vi "ttm_variableSaver_poller.vi"   [LabVIEW 2010]
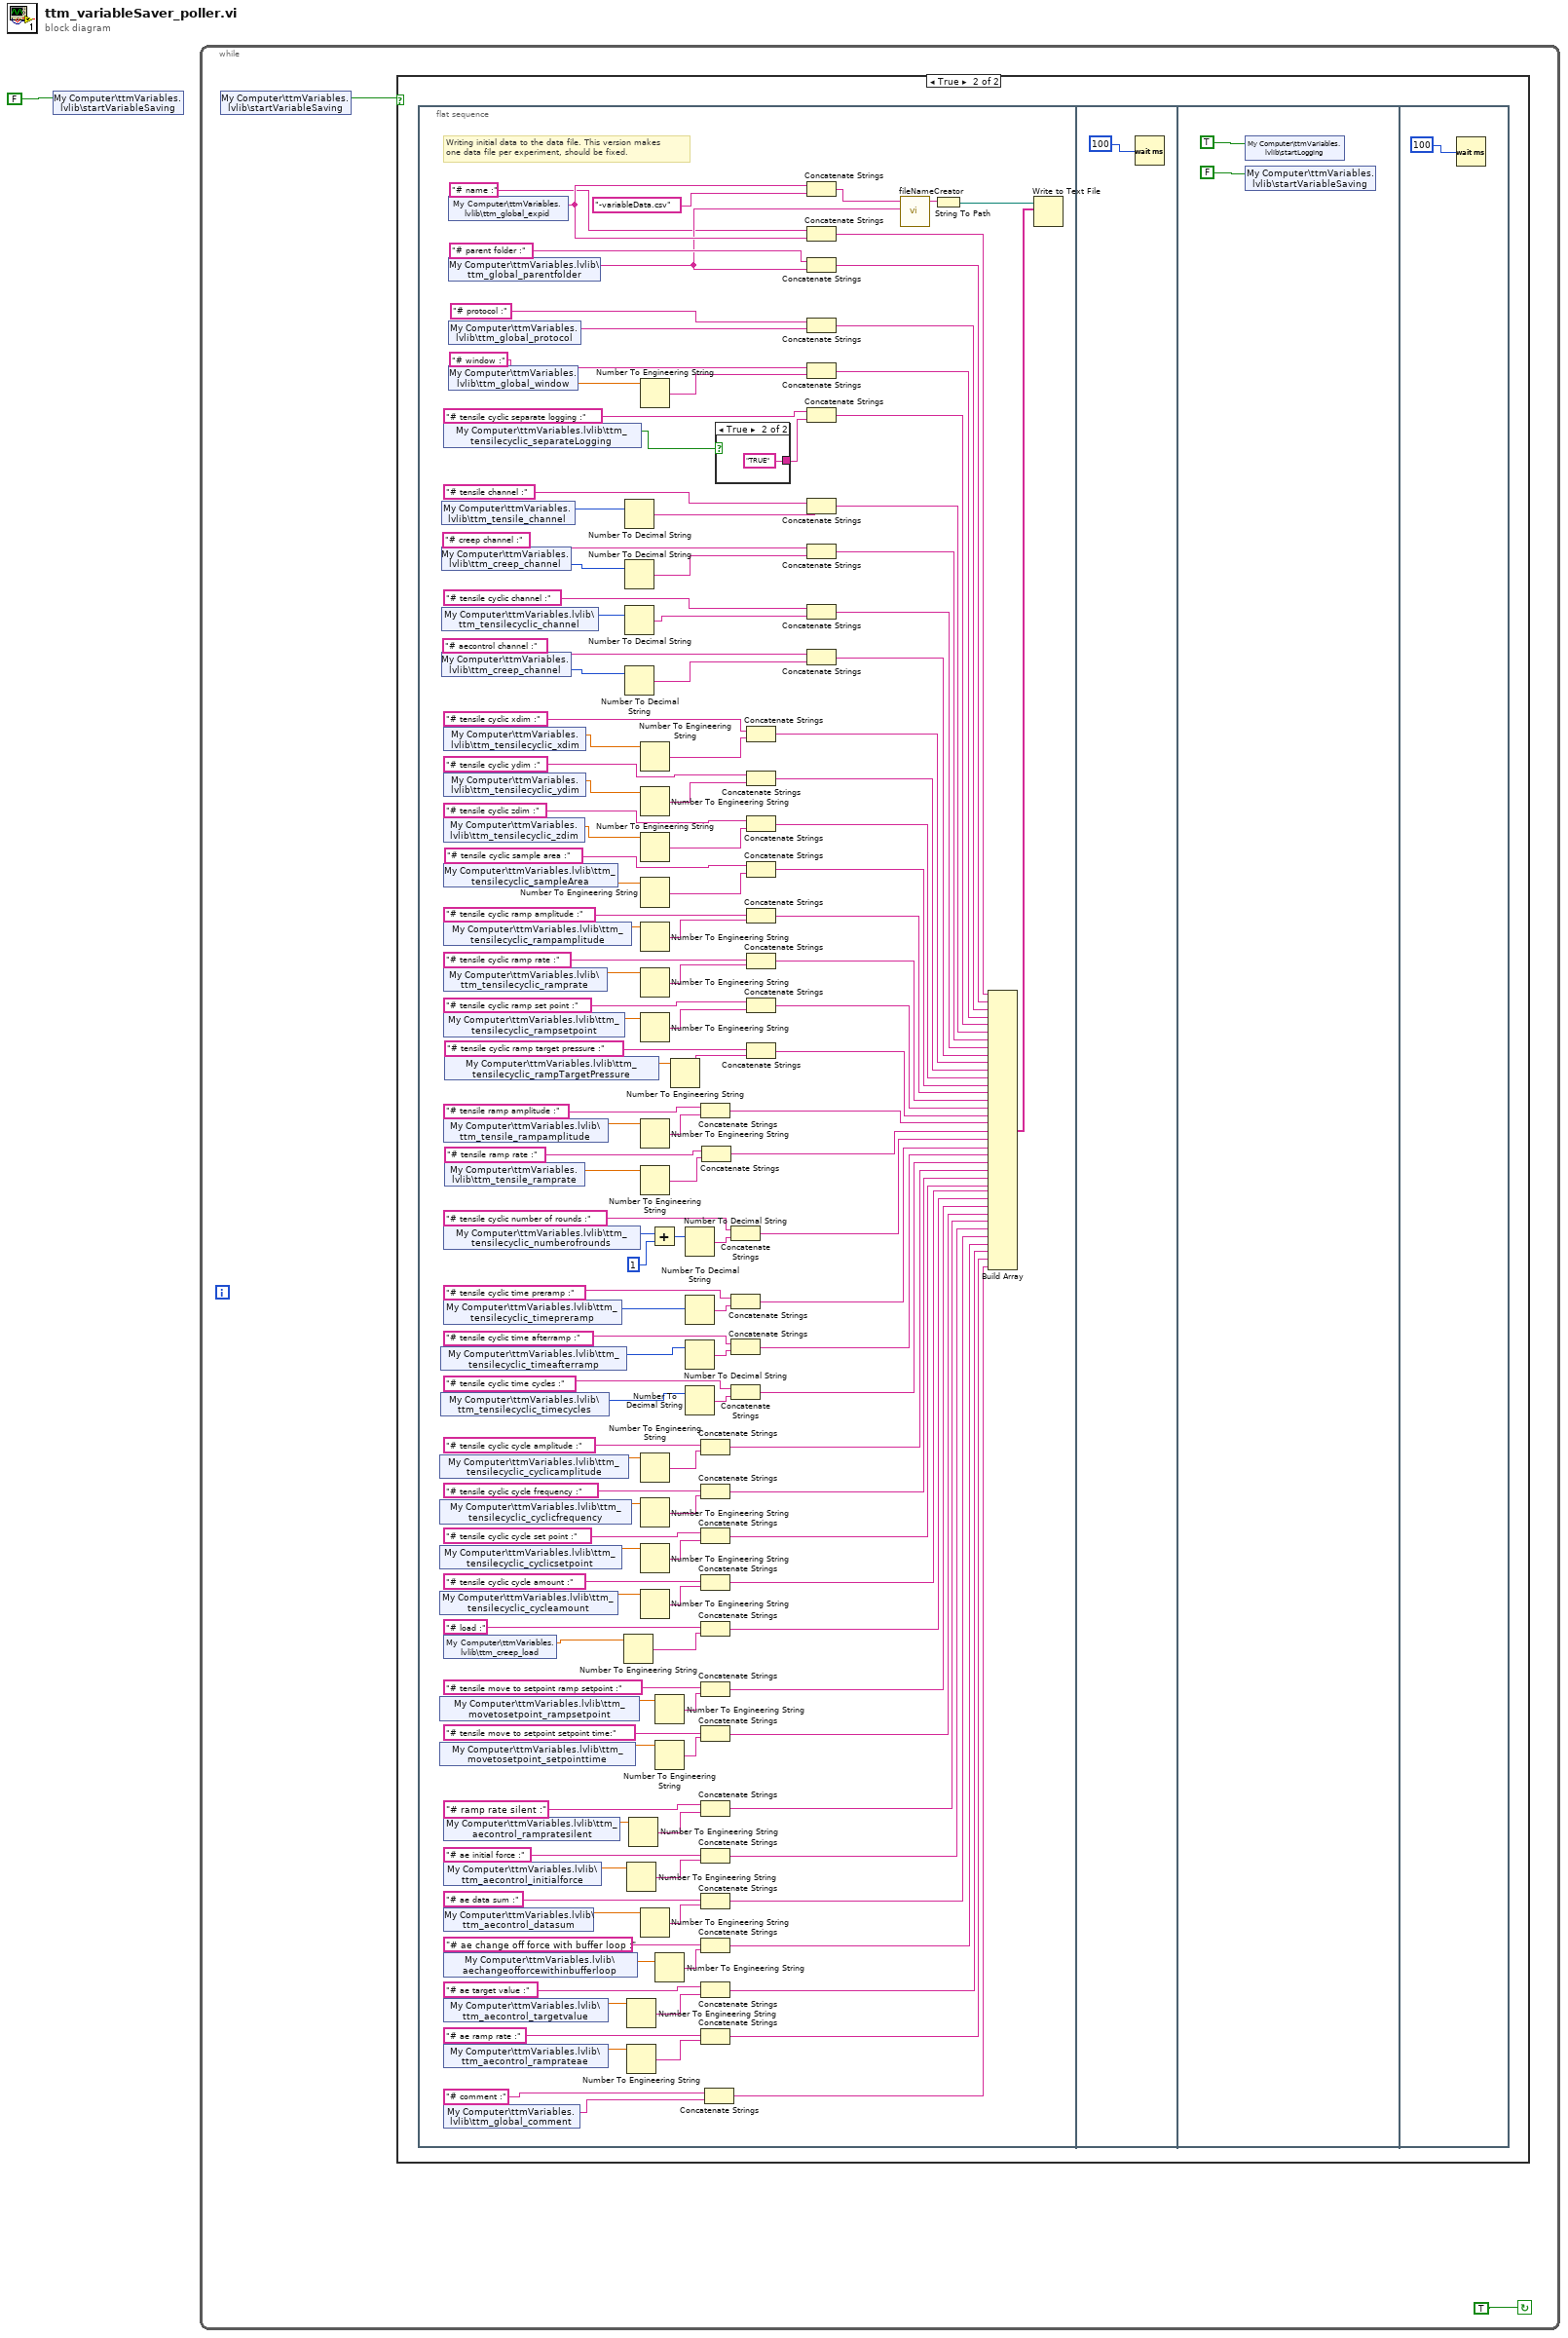
[diagram p0: block diagram]
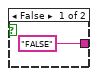
[diagram p3: hidden frame]
diagram:
  n1 = shared-variable "My Computer\\ttmVariables.lvlib\\startVariableSaving"(FALSE ("startLogging")) -> ()  [unwired: 1 in, 1 out]
  n2 = while {
    stop <- TRUE continue-if-true
    n3 = shared-variable "My Computer\\ttmVariables.lvlib\\startVariableSaving"() -> (w2:bool)  [unwired: 1 in, 1 out]
    n4 = case shown="True" w2 {
      frame False {
      }
      frame True {
        n5 = flat-sequence {
          frame #0 {
            # "Writing initial data to the data file. This version makes\none data file per experiment, should be fixed."
            n6 = shared-variable "My Computer\\ttmVariables.lvlib\\ttm_tensilecyclic_cyclicamplitude"() -> (w80:dbl)  [unwired: 1 in, 1 out]
            n7 = shared-variable "My Computer\\ttmVariables.lvlib\\ttm_tensilecyclic_cyclicfrequency"() -> (w81:dbl)  [unwired: 1 in, 1 out]
            n8 = shared-variable "My Computer\\ttmVariables.lvlib\\ttm_tensilecyclic_cyclicsetpoint"() -> (w82:dbl)  [unwired: 1 in, 1 out]
            n9 = shared-variable "My Computer\\ttmVariables.lvlib\\ttm_tensilecyclic_cycleamount"() -> (w83:dbl)  [unwired: 1 in, 1 out]
            n10 = shared-variable "My Computer\\ttmVariables.lvlib\\ttm_movetosetpoint_rampsetpoint"() -> (w13:dbl)  [unwired: 1 in, 1 out]
            n11 = shared-variable "My Computer\\ttmVariables.lvlib\\ttm_movetosetpoint_setpointtime"() -> (w14:dbl)  [unwired: 1 in, 1 out]
            n12 = shared-variable "My Computer\\ttmVariables.lvlib\\ttm_tensilecyclic_timeafterramp"() -> (w78:i32)  [unwired: 1 in, 1 out]
            n13 = shared-variable "My Computer\\ttmVariables.lvlib\\ttm_tensilecyclic_timecycles"() -> (w79:i32)  [unwired: 1 in, 1 out]
            n14 = shared-variable "My Computer\\ttmVariables.lvlib\\ttm_tensile_channel"() -> (w57:i32)  [unwired: 1 in, 1 out]
            n15 = shared-variable "My Computer\\ttmVariables.lvlib\\ttm_creep_channel"() -> (w59:i32)  [unwired: 1 in, 1 out]
            n16 = shared-variable "My Computer\\ttmVariables.lvlib\\ttm_tensilecyclic_channel"() -> (w50:i32)  [unwired: 1 in, 1 out]
            n17 = shared-variable "My Computer\\ttmVariables.lvlib\\ttm_creep_channel"() -> (w52:i32)  [unwired: 1 in, 1 out]
            n18 = shared-variable "My Computer\\ttmVariables.lvlib\\ttm_tensilecyclic_separateLogging"() -> (w63:bool)  [unwired: 1 in, 1 out]
            n19 = shared-variable "My Computer\\ttmVariables.lvlib\\ttm_tensilecyclic_xdim"() -> (w84:dbl)  [unwired: 1 in, 1 out]
            n20 = shared-variable "My Computer\\ttmVariables.lvlib\\ttm_tensilecyclic_ydim"() -> (w85:dbl)  [unwired: 1 in, 1 out]
            n21 = shared-variable "My Computer\\ttmVariables.lvlib\\ttm_tensilecyclic_zdim"() -> (w86:dbl)  [unwired: 1 in, 1 out]
            n22 = shared-variable "My Computer\\ttmVariables.lvlib\\ttm_tensilecyclic_sampleArea"() -> (w152:dbl)  [unwired: 1 in, 1 out]
            n23 = shared-variable "My Computer\\ttmVariables.lvlib\\ttm_tensilecyclic_rampamplitude"() -> (w74:dbl)  [unwired: 1 in, 1 out]
            n24 = shared-variable "My Computer\\ttmVariables.lvlib\\ttm_tensilecyclic_ramprate"() -> (w75:dbl)  [unwired: 1 in, 1 out]
            n25 = shared-variable "My Computer\\ttmVariables.lvlib\\ttm_tensilecyclic_rampsetpoint"() -> (w76:dbl)  [unwired: 1 in, 1 out]
            n26 = shared-variable "My Computer\\ttmVariables.lvlib\\ttm_tensile_rampamplitude"() -> (w44:dbl)  [unwired: 1 in, 1 out]
            n27 = shared-variable "My Computer\\ttmVariables.lvlib\\ttm_tensilecyclic_numberofrounds"() -> (w20:i32)  [unwired: 1 in, 1 out]
            n28 = shared-variable "My Computer\\ttmVariables.lvlib\\ttm_tensilecyclic_timepreramp"() -> (w77:i32)  [unwired: 1 in, 1 out]
            n29 = shared-variable "My Computer\\ttmVariables.lvlib\\ttm_creep_load"() -> (w122:dbl)  [unwired: 1 in, 1 out]
            n30 = shared-variable "My Computer\\ttmVariables.lvlib\\ttm_aecontrol_rampratesilent"() -> (w123:dbl)  [unwired: 1 in, 1 out]
            n31 = shared-variable "My Computer\\ttmVariables.lvlib\\ttm_aecontrol_initialforce"() -> (w133:dbl)  [unwired: 1 in, 1 out]
            n32 = shared-variable "My Computer\\ttmVariables.lvlib\\ttm_aecontrol_datasum"() -> (w134:dbl)  [unwired: 1 in, 1 out]
            n33 = shared-variable "My Computer\\ttmVariables.lvlib\\aechangeofforcewithinbufferloop"() -> (w135:dbl)  [unwired: 1 in, 1 out]
            n34 = shared-variable "My Computer\\ttmVariables.lvlib\\ttm_aecontrol_targetvalue"() -> (w136:dbl)  [unwired: 1 in, 1 out]
            n35 = shared-variable "My Computer\\ttmVariables.lvlib\\ttm_aecontrol_ramprateae"() -> (w137:dbl)  [unwired: 1 in, 1 out]
            n36 = shared-variable "My Computer\\ttmVariables.lvlib\\ttm_global_comment"() -> (w121:string)  [unwired: 1 in, 1 out]
            n37 = shared-variable "My Computer\\ttmVariables.lvlib\\ttm_tensilecyclic_rampTargetPressure"() -> (w149:dbl)  [unwired: 1 in, 1 out]
            n38 = shared-variable "My Computer\\ttmVariables.lvlib\\ttm_tensile_ramprate"() -> (w47:dbl)  [unwired: 1 in, 1 out]
            n39 = shared-variable "My Computer\\ttmVariables.lvlib\\ttm_global_expid"() -> (w90:string)  [unwired: 1 in, 1 out]
            n40 = shared-variable "My Computer\\ttmVariables.lvlib\\ttm_global_parentfolder"() -> (w66:string)  [unwired: 1 in, 1 out]
            n41 = shared-variable "My Computer\\ttmVariables.lvlib\\ttm_global_protocol"() -> (w129:string)  [unwired: 1 in, 1 out]
            n42 = shared-variable "My Computer\\ttmVariables.lvlib\\ttm_global_window"() -> (w131:dbl)  [unwired: 1 in, 1 out]
            n43 = Number To Engineering String(4:w122) -> (0:w125:string)  [unwired: 3 in]
            n44 = Number To Decimal String(number=w57) -> (decimal integer string=w58:string)  [unwired: 1 in]
            n45 = Number To Decimal String(number=w59) -> (decimal integer string=w60:string)  [unwired: 1 in]
            n46 = Number To Decimal String(number=w50) -> (decimal integer string=w51:string)  [unwired: 1 in]
            n47 = Number To Decimal String(number=w52) -> (decimal integer string=w53:string)  [unwired: 1 in]
            n48 = Number To Engineering String(4:w133) -> (0:w139:string)  [unwired: 3 in]
            n49 = Number To Engineering String(4:w136) -> (0:w145:string)  [unwired: 3 in]
            n50 = Number To Engineering String(4:w137) -> (0:w147:string)  [unwired: 3 in]
            n51 = Number To Engineering String(4:w123) -> (0:w127:string)  [unwired: 3 in]
            n52 = Number To Engineering String(4:w131) -> (0:w132:string)  [unwired: 3 in]
            n53 = Number To Engineering String(4:w84) -> (0:w91:string)  [unwired: 3 in]
            n54 = Number To Engineering String(4:w85) -> (0:w94:string)  [unwired: 3 in]
            n55 = Number To Engineering String(4:w86) -> (0:w96:string)  [unwired: 3 in]
            n56 = Number To Engineering String(4:w152) -> (0:w154:string)  [unwired: 3 in]
            n57 = Number To Engineering String(4:w74) -> (0:w98:string)  [unwired: 3 in]
            n58 = Number To Engineering String(4:w75) -> (0:w100:string)  [unwired: 3 in]
            n59 = Number To Engineering String(4:w76) -> (0:w102:string)  [unwired: 3 in]
            n60 = Number To Engineering String(4:w44) -> (0:w46:string)  [unwired: 3 in]
            n61 = Number To Engineering String(4:w47) -> (0:w49:string)  [unwired: 3 in]
            n62 = Number To Engineering String(4:w80) -> (0:w112:string)  [unwired: 3 in]
            n63 = Number To Engineering String(4:w81) -> (0:w114:string)  [unwired: 3 in]
            n64 = Number To Engineering String(4:w82) -> (0:w116:string)  [unwired: 3 in]
            n65 = Number To Engineering String(4:w83) -> (0:w118:string)  [unwired: 3 in]
            n66 = Number To Engineering String(4:w134) -> (0:w141:string)  [unwired: 3 in]
            n67 = Add(x=w20, y=1) -> (x+y=w19:i32)
            n68 = Number To Engineering String(4:w13) -> (0:w16:string)  [unwired: 3 in]
            n69 = Number To Engineering String(4:w14) -> (0:w18:string)  [unwired: 3 in]
            n70 = Number To Engineering String(4:w135) -> (0:w143:string)  [unwired: 3 in]
            n71 = Number To Engineering String(4:w149) -> (0:w151:string)  [unwired: 3 in]
            n72 = Number To Decimal String(number=w19) -> (decimal integer string=w104:string)  [unwired: 1 in]
            n73 = Number To Decimal String(number=w77) -> (decimal integer string=w106:string)  [unwired: 1 in]
            n74 = Number To Decimal String(number=w78) -> (decimal integer string=w108:string)  [unwired: 1 in]
            n75 = Number To Decimal String(number=w79) -> (decimal integer string=w110:string)  [unwired: 1 in]
            n76 = Concatenate Strings("# tensile ramp amplitude :", w46) -> (w33:string)
            n77 = Concatenate Strings("# tensile cyclic cycle amplitude :", w112) -> (w27:string)
            n78 = Concatenate Strings("# tensile cyclic cycle frequency :", w114) -> (w26:string)
            n79 = Concatenate Strings("# tensile cyclic cycle set point :", w116) -> (w25:string)
            n80 = Concatenate Strings("# tensile cyclic cycle amount :", w118) -> (w24:string)
            n81 = Concatenate Strings("# load :", w125) -> (w23:string)
            n82 = Concatenate Strings("# tensile move to setpoint ramp setpoint :", w16) -> (w11:string)
            n83 = Concatenate Strings("# tensile move to setpoint setpoint time:", w18) -> (w10:string)
            n84 = Concatenate Strings("# ramp rate silent :", w127) -> (w9:string)
            n85 = Concatenate Strings("# ae initial force :", w139) -> (w4:string)
            n86 = Concatenate Strings("# ae data sum :", w141) -> (w5:string)
            n87 = Concatenate Strings("# ae change off force with buffer loop :", w143) -> (w6:string)
            n88 = Concatenate Strings("# ae target value :", w145) -> (w7:string)
            n89 = Concatenate Strings("# ae ramp rate :", w147) -> (w8:string)
            n90 = Concatenate Strings("# tensile ramp rate :", w49) -> (w32:string)
            n91 = Concatenate Strings("# comment :", w121) -> (w12:string)
            n92 = case shown="True" w63 {
              tunnel: ["FALSE" "TRUE"] -> w64
              frame False {
              }
              frame True {
              }
            }
            n93 = Concatenate Strings("# tensile cyclic number of rounds :", w104) -> (w31:string)
            n94 = Concatenate Strings("# tensile cyclic time preramp :", w106) -> (w30:string)
            n95 = Concatenate Strings("# tensile cyclic time afterramp :", w108) -> (w29:string)
            n96 = Concatenate Strings("# tensile cyclic time cycles :", w110) -> (w28:string)
            n97 = Concatenate Strings("# tensile cyclic xdim :", w91) -> (w41:string)
            n98 = Concatenate Strings("# tensile cyclic ydim :", w94) -> (w40:string)
            n99 = Concatenate Strings("# tensile cyclic zdim :", w96) -> (w39:string)
            n100 = Concatenate Strings("# tensile cyclic sample area :", w154) -> (w38:string)
            n101 = Concatenate Strings("# tensile cyclic ramp amplitude :", w98) -> (w37:string)
            n102 = Concatenate Strings("# tensile cyclic ramp rate :", w100) -> (w36:string)
            n103 = Concatenate Strings("# tensile cyclic ramp set point :", w102) -> (w35:string)
            n104 = Concatenate Strings("# tensile cyclic ramp target pressure :", w151) -> (w34:string)
            n105 = Concatenate Strings(w90, "-variableData.csv") -> (w89:string)
            n106 = Concatenate Strings("# name :", w90) -> (w71:string)
            n107 = Concatenate Strings("# parent folder :", w66) -> (w70:string)
            n108 = Concatenate Strings("# protocol :", w129) -> (w69:string)
            n109 = Concatenate Strings("# window :", w132) -> (w68:string)
            n110 = Concatenate Strings("# tensile cyclic separate logging :", w64) -> (w67:string)
            n111 = Concatenate Strings("# tensile channel :", w58) -> (w56:string)
            n112 = Concatenate Strings("# creep channel :", w60) -> (w22:string)
            n113 = Concatenate Strings("# tensile cyclic channel :", w51) -> (w43:string)
            n114 = Concatenate Strings("# aecontrol channel :", w53) -> (w42:string)
            n115 = call "fileNameCreator.vi"("folder"=w66, "Measurement ID"=w89) -> ("concatenated string"=w72:string)  [unwired: 9 in]
            n116 = String To Path(string=w72) -> (path=w73:path)
            n117 = Build Array(w71, w70, w69, w68, w67, w56, w22, w43, w42, w41, w40, w39, w38, w37, w36, w35, w34, w33, w32, w31, w30, w29, w28, w27, w26, w25, w24, w23, w11, w10, w9, w4, w5, w6, w7, w8, w12) -> (w87:string[])
            n118 = Write to Text File(file (use dialog)=w73, text=w87) -> ()  [unwired: 2 in, 3 out]
          }
          frame #1 {
            n119 = Wait (ms)(milliseconds to wait=u32 100) -> ()  [unwired: 1 out]
          }
          frame #2 {
            n120 = shared-variable "My Computer\\ttmVariables.lvlib\\startLogging"(TRUE ("startLogging")) -> ()  [unwired: 1 in, 1 out]
            n121 = shared-variable "My Computer\\ttmVariables.lvlib\\startVariableSaving"(FALSE ("startLogging")) -> ()  [unwired: 1 in, 1 out]
          }
          frame #3 {
            n122 = Wait (ms)(milliseconds to wait=u32 100) -> ()  [unwired: 1 out]
          }
        }
      }
    }
  }
